vi "Read Other Images.vi"(8 "error in (no error)":errorcluster, 11 "ParseVectorFile in":refnum<class "ParseVectorFile.lvclass">) -> (0 "error out":errorcluster, 2 "Other Images":refnum<class "SVGImage.lvclass">[](array[class]), 3 "ParseVectorFile out":refnum<class "ParseVectorFile.lvclass">)   [LabVIEW 2019, in "ParseVectorFile.lvclass"]
uses:
  ParseVectorFile.lvclass
  Image/SVGImage.lvclass
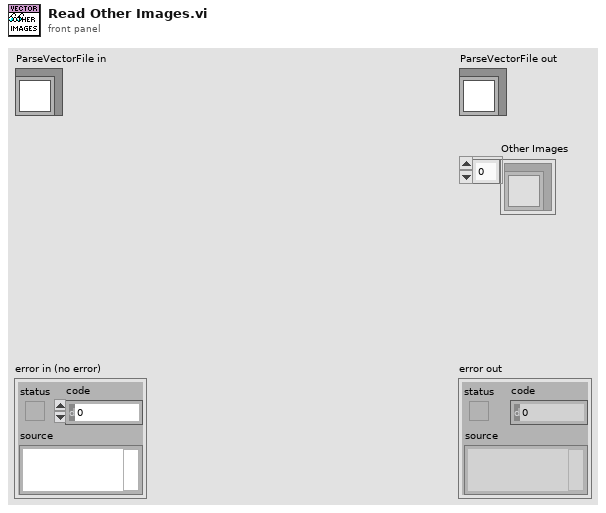
[diagram p1: front panel]
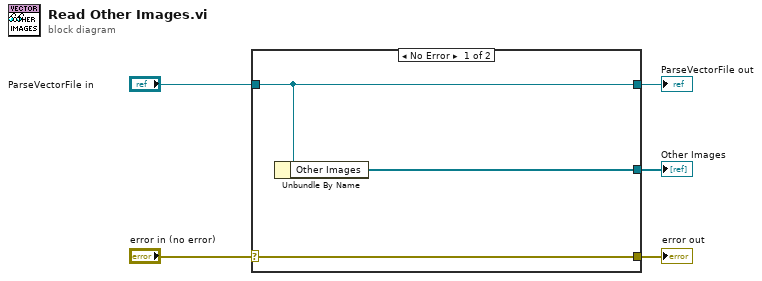
[diagram p0: block diagram]
diagram:
  n1 = case shown="No Error" "error in (no error)" {
    selector: "error in (no error)" -> [w8 w9]
    tunnel: [w8 w9] -> w4
    tunnel: [w7 w10] -> w2
    tunnel: "ParseVectorFile in" -> [w7 w10]
    tunnel: [w6 _] -> w1
    frame No Error {
      n2 = Unbundle By Name(w7) -> ("Other Images"=w6:refnum<class "SVGImage.lvclass">[])
    }
    frame Error {
    }
  }
  "error out" <- w4
  "ParseVectorFile out" <- w2
  "Other Images" <- w1
